vi "_ring_enum_builder.vi"() -> ()   [LabVIEW 2023]
panel:
  in  "data":u16(ring)=102 items=["1D Example Data"=100, "-"=101, "Doppler"=102, "HOP"=103, "TF Sine"=104, "Noisy Doppler"=105, "Sea Temperature"=106, "Sp500"=107, "Power Line"=108, "Engine Knocking"=109, "HeaviSine"=110, "Bumps"=111, "Blocks"=112, "Piece Regular"=113, "HypChirps"=114, "LinChirps"=115, "Chirps"=116, "Piece Polynomial"=117, "ECG"=131, "-"=118, "2D Example Data"=119, "-"=120, "Finger Print (Image)"=121, "Iris Flower (Image)"=122, "Mammogram (Image)"=123, "Lake (Image)"=127, "Two Can 1 (Image)"=132, "Two Can 2 (Image)"=133, "Camera Man (Image)"=134]
  out "array":string[](array[string])
  out "String":string
  out "Array":string[](array[string])
  in  "Enum":T1(ring)
  in  "Text Ring":u16(ring) items=["Balls2", "Battery1", "Battery2", "Connector1", "Subwoofer1", "Subwoofer2", "Subwoofer3", "Subwoofer4", "Hase1", "Lamp1", "Lamp2", "Mouse1", "PhotoLens1", "Po1", "PowerSupply1", "Router", "-", "Stepwedge1", "Stepwedge2", "Stepwedge3", "-", "Fusion160kV", "Fusion2-120kV", "Fusion2-320kV", "Fusion300kV", "FusionPart1-120kV", "FusionPart1-180kV", "-", "Part1", "Part2", "Part3", "Part4", "Part5", "Part6", "Part7", "Part8", "-", "Step2737-02Int", "Step2737-04Int", "Step2737-08Int", "Step2737-16Int", "Step2737-32Int", "Step2737-64Int"]
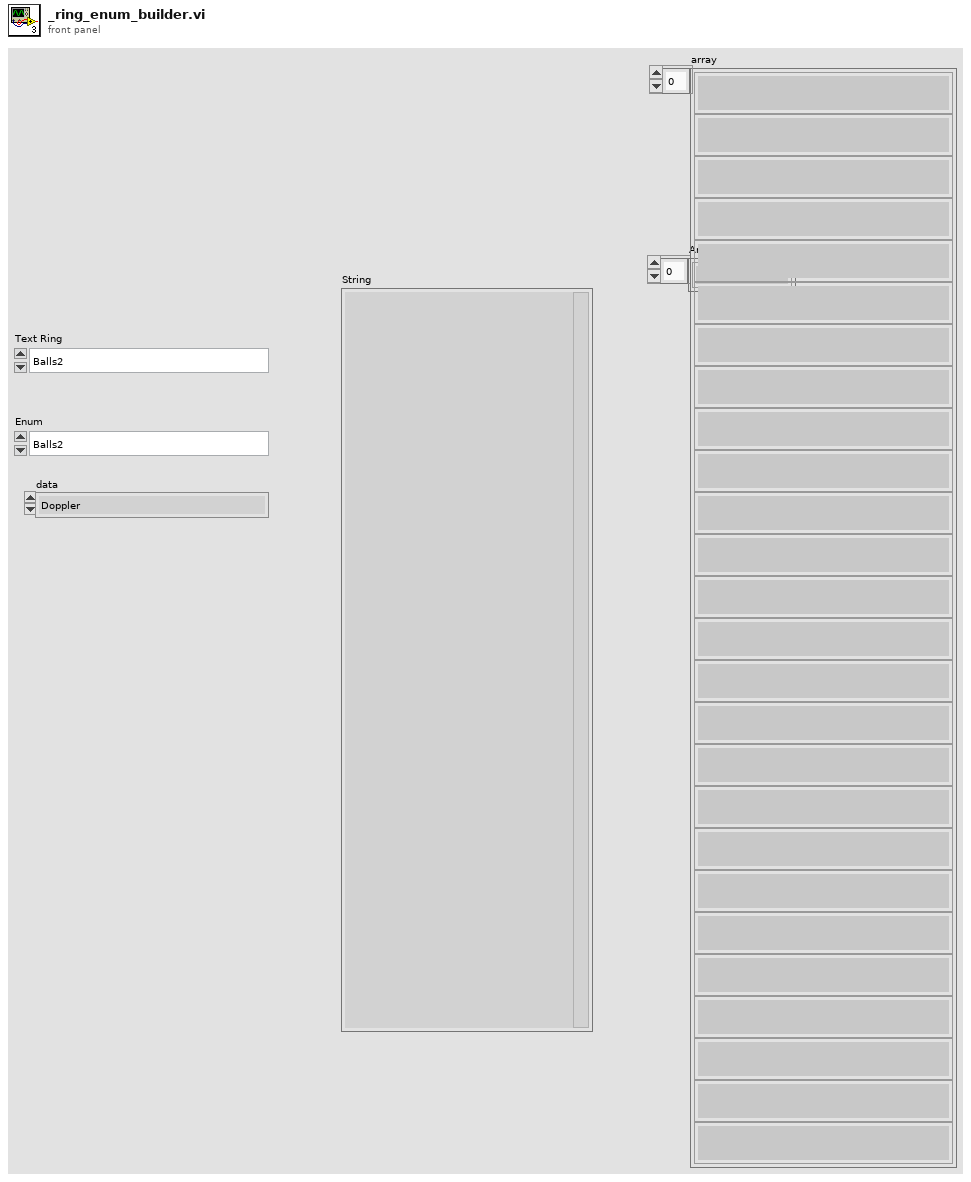
[diagram p1: front panel]
types:
  T1 = enum16{"Balls2", "Battery1", "Battery2", "Connector1", "Fusion160kV", "Fusion2-120kV", "Fusion2-320kV", "Fusion300kV", "Hase1", "Lamp1", "Lamp2", "Mouse1", "Part1", "Part2", "Part3", "Part4", "Part5", "Part6", "Part7", "Part8", "PhotoLens1", "Po1", "PowerSupply1", "Router", "Step2737-02Int", "Step2737-04Int", "Step2737-08Int", "Step2737-16Int", "Step2737-32Int", "Step2737-64Int", "Stepwedge1", "Stepwedge2", "Stepwedge3", "Subwoofer1", "Subwoofer2", "Subwoofer3", "Subwoofer4"}
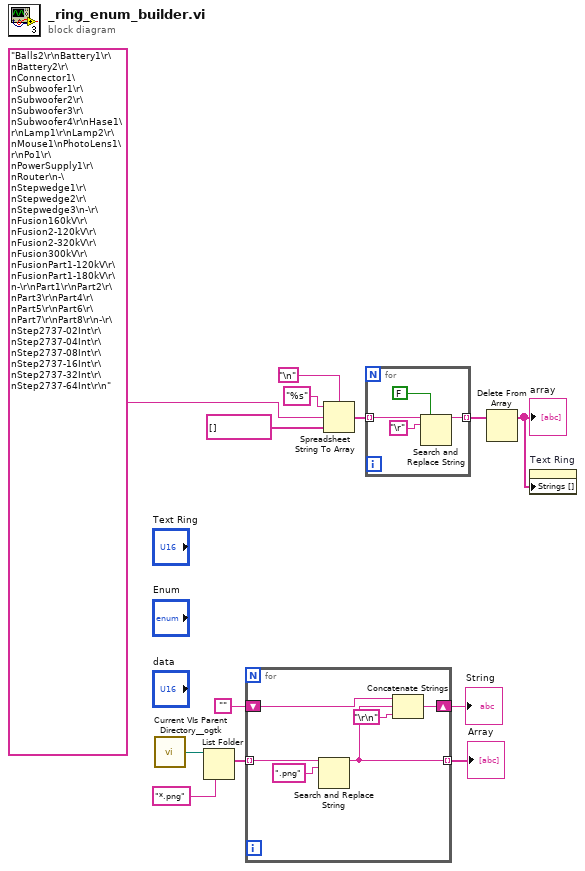
[diagram p0: block diagram]
diagram:
  n1 = call <userlib>:"Current VIs Parent Directory__ogtk.vi"() -> ("Parent Directory (+ Relative)"=w13:path)  [unwired: 5 in]
  n2 = List Folder(path=w13, pattern="*.png") -> (filenames=w11:string[])  [unwired: 2 in, 3 out]
  n3 = for {
    tunnel: w11 -> [w19] mode=indexing
    tunnel: [w16] -> w8 mode=indexing
    shift-right: [w14] -> w9
    shift-left: "" -> [w17]
    n4 = Search and Replace String(input string=w19, search string=".png" ("regular expression")) -> (result string=w16:string)  [unwired: 6 in, 3 out]
    n5 = Concatenate Strings(w17, w16, "\r\n") -> (w14:string)
  }
  "Array" <- w8
  "String" <- w9
  n6 = Spreadsheet String To Array(delimiter (Tab)="\n", format string="%s", spreadsheet string="Balls2\r\nBattery1\r\nBattery2\r\nConnector1\nSubwoofer1\r\nSubwoofer2\r\nSubwoofer3\r\nSubwoofer4\r\nHase1\r\nLamp1\r\nLamp2\r\nMouse1\nPhotoLens1\r\nPo1\r\nPowerSupply1\r\nRouter\n-\nStepwedge1\r\nStepwedge2\r\nStepwedge3\n-\r\nFusion160kV\r\nFusion2-120kV\r\nFusion2-320kV\r\nFusion300kV\r\nFusionPart1-120kV\r\nFusionPart1-180kV\r\n-\r\nPart1\r\nPart2\r\nPart3\r\nPart4\r\nPart5\r\nPart6\r\nPart7\r\nPart8\r\n-\r\nStep2737-02Int\r\nStep2737-04Int\r\nStep2737-08Int\r\nStep2737-16Int\r\nStep2737-32Int\r\nStep2737-64Int\r\n" ("String"), array type (2D Dbl)=string[] []) -> (array=w3:string[])
  n7 = for {
    tunnel: w3 -> [w23] mode=indexing
    tunnel: [w20] -> w2 mode=indexing
    n8 = Search and Replace String(replace all?=FALSE ("replace all? (F)"), input string=w23, search string="\r") -> (result string=w20:string)  [unwired: 5 in, 3 out]
  }
  n9 = Delete From Array(array=w2) -> (array with subset deleted=w1:string[])  [unwired: 2 in, 1 out]
  "array" <- w1
  n10 = property on="Text Ring" class="Ring (strict)"("Strings []"=w1) -> ()  [unwired: 2 in, 2 out]
